vi "iq cluster to iq.vi"(0 "data in":T1) -> (4 "i in":fxp<+/-,64,1> format="%.64g", 6 "q in":fxp<+/-,64,1> format="%.64g")   [LabVIEW 2018]
uses:
  <instrlib>/_niInstr/DSP/v1/Shared/Public/IQ Data.ctl
  <instrlib>/_niInstr/DSP/v1/Shared/niInstr DSP v1 Shared.lvlib
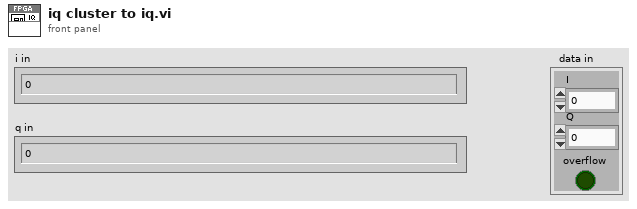
[diagram p1: front panel]
types:
  T1 = typedef "niInstr DSP v1 Shared.lvlib/IQ Data.ctl" = cluster{"I":fxp<+/-,18,1>, "Q":fxp<+/-,18,1>, "overflow":bool}
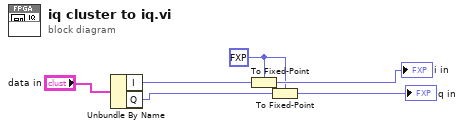
[diagram p0: block diagram]
diagram:
  w1 = fxp<+/-,64,1> 0.0 ("i in")
  n1 = Unbundle By Name("data in") -> ("I"=w5:fxp<+/-,18,1>, "Q"=w4:fxp<+/-,18,1>)
  n2 = To Fixed-Point(fixed-point type=w1, number=w5) -> (fixed-point=→"i in":fxp<+/-,64,1>)
  n3 = To Fixed-Point(fixed-point type=w1, number=w4) -> (fixed-point=→"q in":fxp<+/-,64,1>)
